vi "Get All Temp (SubVI).vi"(10 "Instrument Type":i32, 11 ".NET引用句柄输入":refnum<k24>) -> (3 "Temperature":dbl)   [LabVIEW 2019, in "SubVI.lvlib"]
uses:
  SubVI.lvlib
  lib/QDInstrument.dll
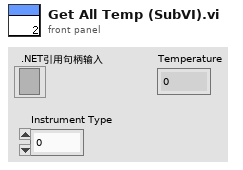
[diagram p1: front panel]
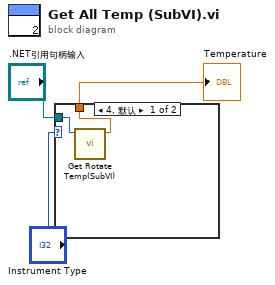
[diagram p0: block diagram]
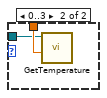
[diagram p2: hidden frame]
diagram:
  n1 = case shown="4, 默认" "Instrument Type" {
    tunnel: [w4 w7] -> w1
    tunnel: ".NET引用句柄输入" -> [w5 w6]
    frame 4, Default {
      n2 = call "Get Rotate Temp(SubVI).vi"(".NET引用句柄输入"=w5) -> ("Result"=w4:dbl)  [unwired: 10 in]
    }
    frame 0..3 {
      n3 = call "GetTemperature.vi"("Instrument Ref In"=w6) -> ("Temperature"=w7:dbl)  [unwired: 4 in, 4 out]
    }
  }
  "Temperature" <- w1
